vi "Populate Devices.vi"(8 "error in (no error)":errorcluster, 10 "List XML File":path, 11 "MCListbox Refnum":refnum<vi>) -> (0 "error out":errorcluster)   [LabVIEW 2013, in "ACNET Devices Editor.lvlib"]
uses:
  ACNET Devices Editor.lvlib
  ACNET Monitor/ACNET Devices.lvclass
  ACNET Monitor/ACNET Device.lvclass
  ACNET Monitor.lvlib
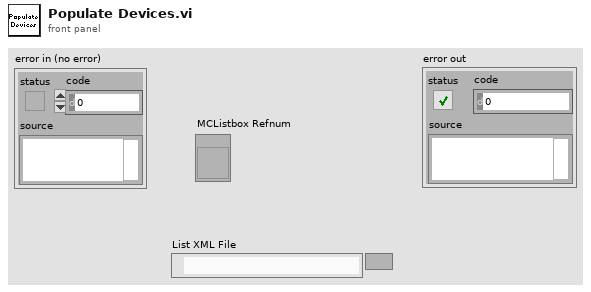
[diagram p1: front panel]
types:
  T1 = cluster{"name":string, "minValue":dbl, "maxValue":dbl, "units":string, "description":string, "ignoreMinValue":bool, "ignoreMaxValue":bool}
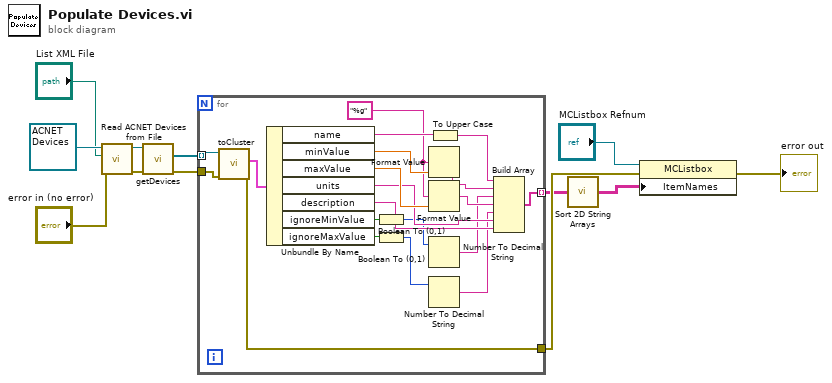
[diagram p0: block diagram]
diagram:
  n1 = call "Read ACNET Devices from File.vi"("error in (no error)"="error in (no error)", "XML File Path"="List XML File", "ACNET Devices in"=refnum<class "ACNET Devices.lvclass"> refnum ("ACNET Device Limits List in")) -> ("error out"=w10:errorcluster, "ACNET Devices out"=w11:refnum<class "ACNET Devices.lvclass">)  [unwired: 6 in, 1 out]
  n2 = call-dynamic "getDevices.vi"("error in (no error)"=w10, "ACNET Devices in"=w11) -> ("error out"=w8:errorcluster, "Devices"=w9:refnum<class "ACNET Device.lvclass">[])  [unwired: 7 in, 1 out]
  n3 = for {
    tunnel: w9 -> [w28] mode=indexing
    tunnel: w8 -> [w29]
    tunnel: [w31] -> w6 mode=indexing
    tunnel: [w27] -> w7
    w23 = "%g" ("format string")
    n4 = call-dynamic "toCluster.vi"("error in (no error)"=w29, "ACNET Device in"=w28) -> ("error out"=w27:errorcluster, "ACNET Device Cluster"=w26:T1)  [unwired: 7 in, 1 out]
    n5 = Unbundle By Name(w26) -> ("name"=w25:string, "minValue"=w24:dbl, "maxValue"=w22:dbl, "units"=w20:string, "description"=w21:string, "ignoreMinValue"=w19:bool, "ignoreMaxValue"=w18:bool)
    n6 = Boolean To (0,1)(Boolean=w19) -> (0, 1=w17:i16)
    n7 = Boolean To (0,1)(Boolean=w18) -> (0, 1=w14:i16)
    n8 = Format Value(format string=w23, value (0)=w24) -> (output string=w32:string)  [unwired: 1 in]
    n9 = Format Value(format string=w23, value (0)=w22) -> (output string=w16:string)  [unwired: 1 in]
    n10 = Number To Decimal String(number=w17) -> (decimal integer string=w15:string)  [unwired: 1 in]
    n11 = Number To Decimal String(number=w14) -> (decimal integer string=w13:string)  [unwired: 1 in]
    n12 = To Upper Case(1:w25) -> (0:w30:string)
    n13 = Build Array(w30, w32, w15, w16, w13, w20, w21) -> (w31:string[])
  }
  n14 = call "Sort 2D String Arrays.vi"("Arrays in"=w6) -> ("Arrays out"=w2:string[][])  [unwired: 4 in]
  n15 = property on="Property Node" class="MCListbox"(reference="MCListbox Refnum", error in=w7, "ItemNames"=w2) -> (error out=→"error out":errorcluster)  [unwired: 1 out]
